vi "MotorTest.vi"() -> ()   [LabVIEW 2019]
uses:
  <vilib>/myRIO/Common/Instrument Driver Framework/myRIO v1.0/Encoder/typedefs/Encoder Count Direction Enum.ctl
  <vilib>/myRIO/Express VI/Onboard IO/Encoder/Encoder Express VI.xnode
  <vilib>/myRIO/Instrument Drivers/Utilities/Utilities.lvlib
  <vilib>/Utility/file.llb/Write Delimited Spreadsheet (DBL).vi
  <vilib>/myRIO/Instrument Drivers/Onboard IO/Encoder/vis/Read.vi
  <vilib>/myRIO/Instrument Drivers/Onboard IO/Encoder/Encoder.lvlib
  <vilib>/myRIO/Common/Instrument Driver Framework/myRIO v1.0/Encoder/typedefs/Encoder Signal Mode.ctl
  <vilib>/myRIO/Common/Instrument Driver Framework/myRIO v1.0/Encoder/typedefs/Encoder Channels Enum.ctl
  <vilib>/myRIO/Common/Instrument Driver Framework/Utilities/typedefs/Generic FPGA Reference.ctl
  <vilib>/myRIO/Common/Instrument Driver Framework/Utilities/typedefs/myRIO v1.0 Reference.ctl
  <vilib>/myRIO/Common/Instrument Driver Framework/Utilities/typedefs/Hardware Version Enum.ctl
  <vilib>/myRIO/Common/Instrument Driver Framework/Utilities/typedefs/myRIO Generic Hardware Reference.ctl
  <vilib>/myRIO/Instrument Drivers/Onboard IO/Encoder/typedefs/Encoder Reference.ctl
  <vilib>/myRIO/Instrument Drivers/Onboard IO/Encoder/vis/myRIO Encoder Open.xnode
  <vilib>/myRIO/Common/Instrument Driver Framework/Utilities/vis/Is FPGA Ref Available.vi
  <vilib>/myRIO/Common/Instrument Driver Framework/myRIO v1.0/Encoder/vis/myRIO v1.1 Open Encoder.vi
  <vilib>/myRIO/Common/Instrument Driver Framework/myRIO v1.0/Encoder/vis/myRIO v1.0 Configure Encoder.vi
  <vilib>/myRIO/Common/Instrument Driver Framework/myRIO v1.0/Encoder/typedefs/Encoder Configuration v1.0.ctl
  <vilib>/userdefined/High Color/nirio_resource_hc.ctl
panel:
  in  "Duty Cycle in":dbl=0.5
  out "error out 2":errorcluster
  in  "Stop 2":bool
  out "Counter Direction":enum16{"Counting Up", "Counting Down"}(ring)
  out "Overflow?":bool
  in  "Reset Counter":bool
  out "actual pos":dbl
  out "Graph 2":cluster{dbl, dbl}(graph)
  in  "Frequency [Hz]":dbl=1000.0
  out "Duty Cycle":dbl=0.5
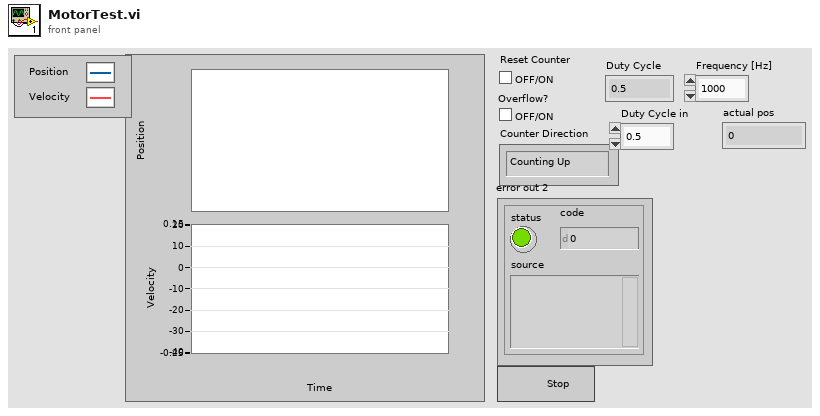
[diagram p1: front panel]
types:
  T1 = typedef "Encoder.lvlib/Encoder Reference.ctl" = cluster{"myRIO Reference":T2, "Encoder Channels Enum":T6}
  T2 = typedef "myRIO Generic Hardware Reference.ctl" = cluster{"myRIO Model":T3, "myRIO Hardware Reference":T4}
  T3 = typedef "Hardware Version Enum.ctl" = enum16{"Unknown", "myRIO-1900", "myRIO-1950", "roboRIO", "NI ELVIS RIO CM", "ELVIS III"}
  T4 = typedef "myRIO v1.0 Reference.ctl" = cluster{"Generic FPGA Reference":T5, "Allow multiple opens":bool}
  T5 = typedef "Generic FPGA Reference.ctl" = refnum<k20>
  T6 = typedef "Encoder Channels Enum.ctl" = enum16{"Not Connected", "C/ENC0", "C/ENC1", "A/ENC", "A/ENC0", "A/ENC1", "A/ENC2", "A/ENC3", "A/ENC4", "A/ENC5", "A/ENC6", "A/ENC7", "A/ENC8", "A/ENC9", "B/ENC", "B/ENC0", "B/ENC1", "B/ENC2", "B/ENC3", "B/ENC4", "B/ENC5", "B/ENC6", "B/ENC7", "B/ENC8", "B/ENC9", "DIO/ENC0", "DIO/ENC1", "DIO/ENC2", "DIO/ENC3", "DIO/ENC4"}
  T7 = typedef "Encoder Signal Mode.ctl" = enum16{"Quadrature phase signal", "Step and direction signal"}
  T8 = typedef "nirio_resource_hc.ctl" = tag
  T9 = typedef "Encoder Count Direction Enum.ctl" = enum16{"Counting Up", "Counting Down"}
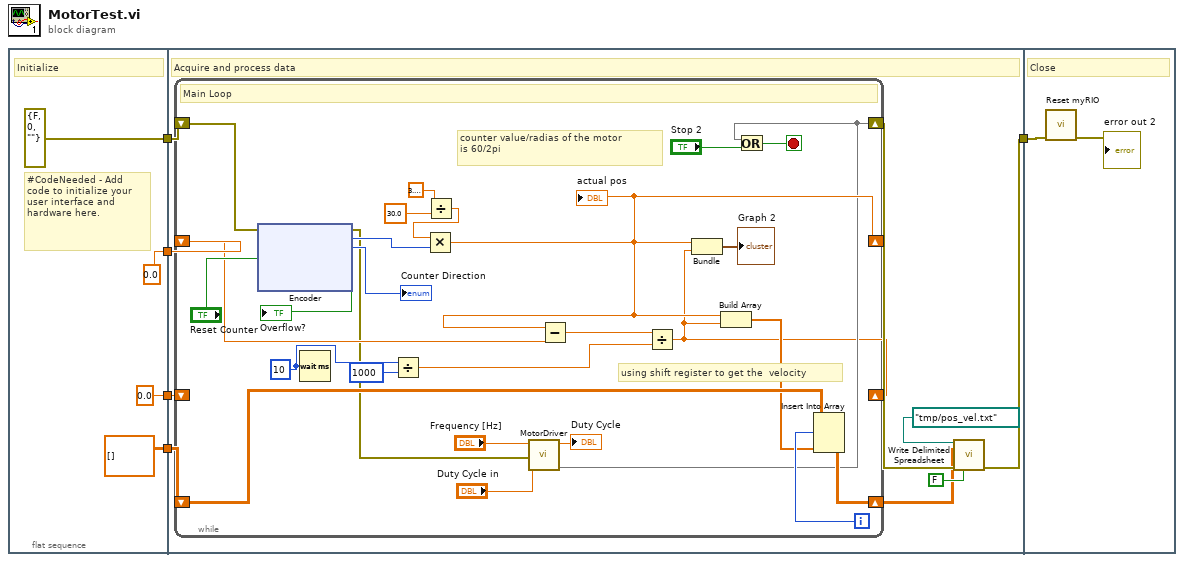
[diagram p0: block diagram]
diagram:
  n1 = flat-sequence {
    tunnel: [errorcluster {"status"=FALSE, "code"=0, "source"=""} ("error in (no error)")] -> w5
    tunnel: [0.0] -> w4
    tunnel: [dbl[][] [] ("array")] -> w3
    tunnel: [0.0] -> w2
    tunnel: w5 -> [w18]
    tunnel: [w13] -> w1
    tunnel: w4 -> [w17]
    tunnel: w3 -> [w16]
    tunnel: w2 -> [w10]
    tunnel: w1 -> [w93]
    frame #0 {
      # "#CodeNeeded - Add code to initialize your user interface and hardware here."
      # "Initialize"
    }
    frame #1 {
      # "Acquire and process data"
      n2 = while {
        shift-right: [w23] -> w14
        shift-left: w18 -> [w19]
        shift-right: [w25] -> _
        shift-left: w17 -> [w38]
        shift-right: [w30] -> w11
        shift-left: w16 -> [w29]
        shift-right: [w22] -> _
        shift-left: w10 -> [_]
        i -> [w31]
        stop <- w44 stop-if-true
        w37 = u32 10 ("milliseconds to wait")
        # "using shift register to get the  velocity"
        # "counter value/radias of the motor \nis 60/2pi"
        # "Main Loop"
        n3 = xnode "Encoder"("Reset Counter"="Reset Counter", "error in (no error)"=w19) -> ("Counter Value"=w34:i32, "Counter Direction"=→"Counter Direction":T9, "Overflow?"=→"Overflow?":bool, "error out"=w24:errorcluster)
        n4 = Wait (ms)(milliseconds to wait=w37) -> ()  [unwired: 1 out]
        n5 = Divide(x=w37, y=u32 1000) -> (x/y=w21:dbl)
        n6 = Divide(x=3.141592653589793, y=30.0) -> (x/y=w33:dbl)
        n7 = Multiply(x=w33, y=w34) -> (x*y=w25:dbl)
        "actual pos" <- w25
        n8 = call "MotorDriver.vi"("error in (no error)"=w24, "Duty Cycle in"="Duty Cycle in", "Frequency [Hz]"="Frequency [Hz]") -> (0:w23, "Duty Cycle out"=→"Duty Cycle":dbl)  [unwired: 7 in]
        n9 = Subtract(x=w25, y=w38) -> (x-y=w35:dbl)
        n10 = Divide(x=w35, y=w21) -> (x/y=w22:dbl)
        n11 = Bundle(w25, w22) -> (→"Graph 2":cluster{dbl, dbl})  [unwired: 1 in]
        n12 = Build Array(w25, w22) -> (w28:dbl[])
        n13 = Or(x=w23, y="Stop 2") -> (x .or. y?=w44:bool)
        n14 = Insert Into Array(array=w29, index (row)=w31, new element=w28) -> (w30:dbl[][])  [unwired: 1 in]
      }
      n15 = call-poly <vilib>:"Write Delimited Spreadsheet.vi"("file path (dialog if empty)"=path "/tmp/pos_vel.txt", "2D data"=w11, "error in (no error)"=w14, "transpose? (no:F)"=FALSE) -> ("error out"=w13:errorcluster)  [unwired: 10 in, 1 out]
    }
    frame #2 {
      # "Close"
      n16 = call <vilib>:"Reset myRIO.vi"("error in (no error)"=w93) -> ("error out"=→"error out 2":errorcluster)  [unwired: 10 in]
    }
  }
